vi "Move piece.vi"(9 "Destination":T1={"File"=enum."a", "Rank"=enum."4"}, 10 "Source":T1={"File"=enum."a", "Rank"=enum."4"}, 11 "Board in":refnum<class "Board.lvclass">) -> (1 "Removed piece":refnum<class "Piece.lvclass">, 2 "Destination occupied?":bool, 3 "Board out":refnum<class "Board.lvclass">)   [LabVIEW 2015, in "Chesslib.lvlib" / "Board.lvclass"]
uses:
  Board.lvclass
  typedef/Square.ctl
  typedef/File.ctl
  typedef/Rank.ctl
  Pieces/Piece/Piece.lvclass
  Chesslib.lvlib
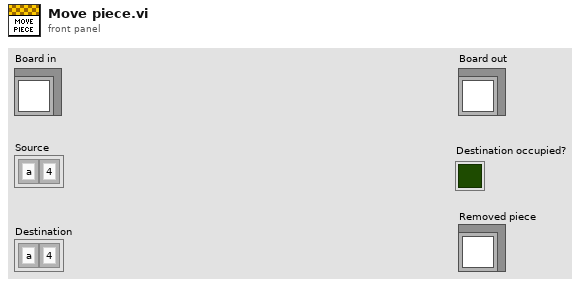
[diagram p1: front panel]
types:
  T1 = typedef "Chesslib.lvlib/Square.ctl" = cluster{"File":T2, "Rank":T3}
  T2 = typedef "Chesslib.lvlib/File.ctl" = enum16{"a", "b", "c", "d", "e", "f", "g", "h"}
  T3 = typedef "Chesslib.lvlib/Rank.ctl" = enum16{"1", "2", "3", "4", "5", "6", "7", "8"}
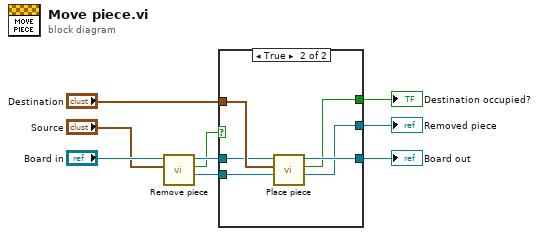
[diagram p0: block diagram]
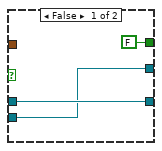
[diagram p2: hidden frame]
diagram:
  n1 = call "Remove piece.vi"("Square"="Source", "Board in"="Board in") -> ("Removed piece"=w2:refnum<class "Piece.lvclass">, "Square occupied?"=w1:bool, "Board out"=w3:refnum<class "Board.lvclass">)  [unwired: 7 in]
  n2 = case shown="True" w1 {
    tunnel: [w12 w18] -> w8
    tunnel: "Destination" -> [_ w17]
    tunnel: [FALSE ("Square occupied?") w16] -> w5
    tunnel: [w11 w15] -> w4
    tunnel: w3 -> [w12 w14]
    tunnel: w2 -> [w11 w13]
    frame False {
    }
    frame True {
      n3 = call "Place piece.vi"("Piece"=w13, "Square"=w17, "Board in"=w14) -> ("Removed piece"=w15:refnum<class "Piece.lvclass">, "Square occupied?"=w16:bool, "Board out"=w18:refnum<class "Board.lvclass">)  [unwired: 6 in]
    }
  }
  "Board out" <- w8
  "Removed piece" <- w4
  "Destination occupied?" <- w5
